vi "Untitled 1.vi"() -> ()   [LabVIEW 2020]
panel:
  out "Waveform Graph":dbl[](graph)
  out "x + iy":cdb[](array[numeric])
  out "size (in bytes)":i64
  out "size(s)":i32
  in  "file path (use dialog)":path
  out "error out":errorcluster
  out "data":i16[](array[numeric])
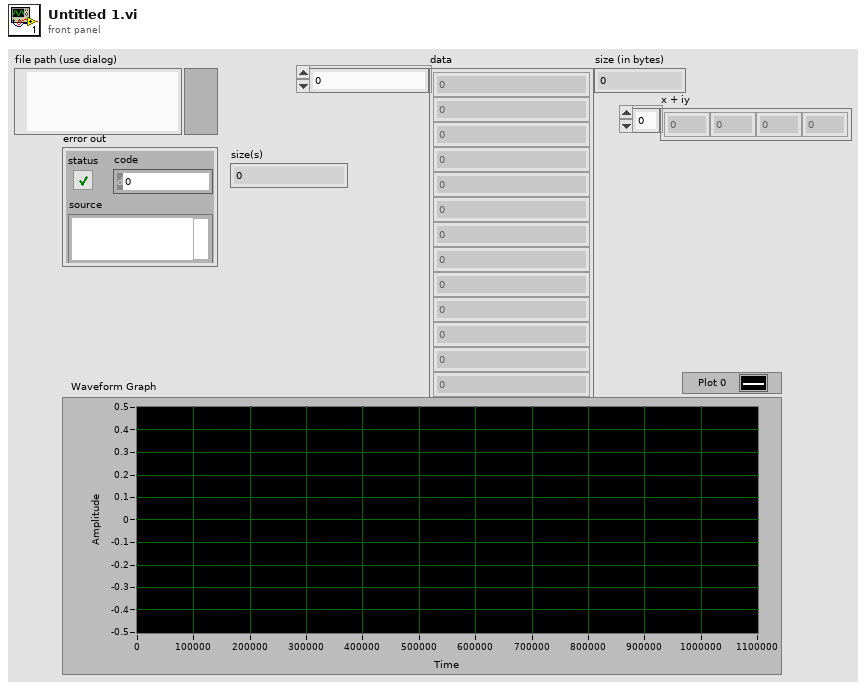
[diagram p1: front panel]
types:
  T1 = enum16{"big-endian, network order", "native, host order", "little-endian"}
  T2 = enum16{"open", "replace", "create", "open or create", "replace or create", "replace or create with confirmation"}
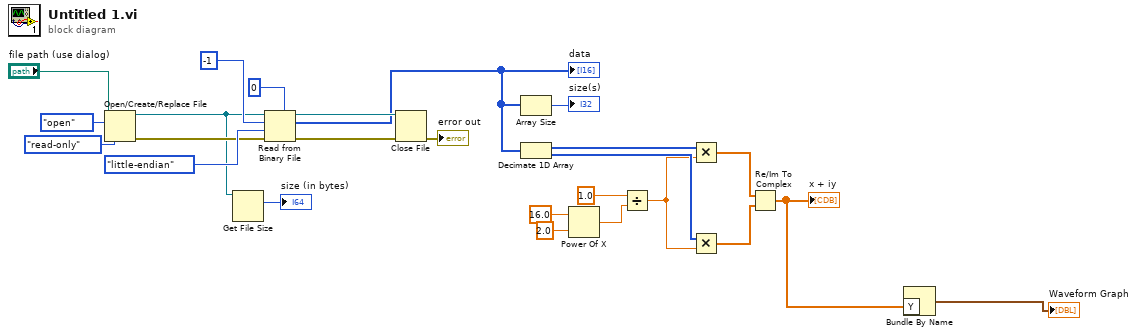
[diagram p0: block diagram]
diagram:
  n1 = Open/Create/Replace File(file path (use dialog)="file path (use dialog)", operation (0:open)=T2."open", access (0:read/write)=enum16{"read/write", "read-only", "write-only"}."read-only") -> (refnum out=w14:refnum<file>, error out=w21:errorcluster)  [unwired: 3 in, 1 out]
  n2 = Get File Size(file=w14) -> (size (in bytes)=→"size (in bytes)":i64)  [unwired: 1 in, 2 out]
  n3 = Read from Binary File(5:i16 0, 8:w21, 9:T1."little-endian" ("byte order (0:big-endian, network order)"), 10:-1 ("count (1)"), 11:w14) -> (0:w18:errorcluster, 2:w12:i16[], 3:w19:refnum<file>)  [unwired: 1 in, 1 out]
  "data" <- w12
  n4 = Close File(refnum=w19, error in=w18) -> (error out=→"error out":errorcluster)  [unwired: 1 out]
  n5 = Array Size(array=w12) -> (size(s)=→"size(s)":i32)
  n6 = Decimate 1D Array(w12) -> (w11:i16[], w10:i16[])
  n7 = Power Of X(1:2.0 ("x"), 2:16.0 ("y")) -> (0:w7:dbl)
  n8 = Divide(x=1.0, y=w7) -> (x/y=w5:dbl)
  n9 = Multiply(x=w11, y=w5) -> (x*y=w4:dbl[])
  n10 = Multiply(x=w10, y=w5) -> (x*y=w3:dbl[])
  n11 = Re/Im To Complex(1:w3, 2:w4) -> (0:w2:cdb[])
  "x + iy" <- w2
  n12 = Bundle By Name("Y"=w2) -> (→"Waveform Graph":waveform(cdb))  [unwired: 1 in]
